vi "WPI_CameraSend Images To PC LoopCustom2.vi"(8 "error in (no error)":errorcluster, 11 "CameraDevRef":T1) -> ()   [LabVIEW 2015]
doc: "This VI is used to send images to the dashboard using the second enet port on the 8 slot controller. This is provided for compatibility, but is higher overhead than using the Camera MJPG approach.\n\nThis software is licensed. Open the labview\\readme\\WPI Robotics Library Open Source License.txt file for more information."
uses:
  <vilib>/Rock Robotics/WPI/Camera/WPI_CameraDevRef.ctl
  <vilib>/Rock Robotics/SystemInterfaces/NetworkCommunication/NetComm_UsageReport_ResourceType.ctl
  Robot Global Data.vi
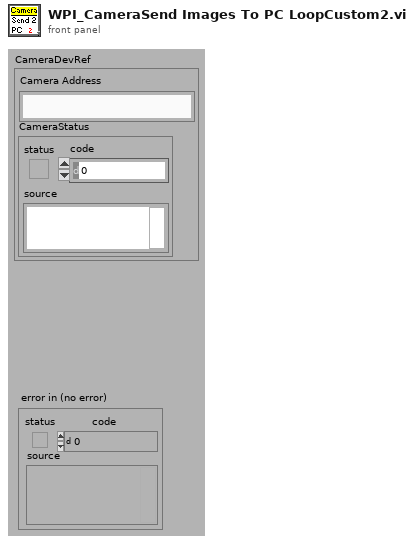
[diagram p1: front panel]
types:
  T1 = typedef "WPI_CameraDevRef.ctl" = cluster{"Camera Address":string, "CameraStatus":errorcluster}
  T2 = cluster{"fps":i32, "compression":i32, "compression 2":i32}
  T3 = typedef "NetComm_UsageReport_ResourceType.ctl" = enum8{"Controller", "Module", "Language", "CANPlugin", "Accelerometer", "ADXL345", "AnalogChannel", "AnalogTrigger", "AnalogTriggerOutput", "CANJaguar", "Compressor", "Counter", "Dashboard", "DigitalInput", "DigitalOutput", "DriverStationCIO", "DriverStationEIO", "DriverStationLCD", "Encoder", "GearTooth", "Gyro", "I2C", "Framework", "Jaguar", "Joystick", "Kinect", "KinectStick", "PIDController", "Preferences", "PWM", "Relay", "RobotDrive", "SerialPort", "Servo", "Solenoid", "SPI", "Task", "Ultrasonic", "Victor", "Button", "Command", "AxisCamera", "PCVideoServer", "SmartDashboard", "Talon", "HiTechnicColorSensor", "HiTechnicAccel", "HiTechnicCompass", "SRF08", "AnalogOutput", "Victor SP", "Talon SRX", "CAN Talon SRX", "ADXL362 Accel", "ADXRS450 Gyro", "Rev SPARK", "Mindsensors SD540", "Digital Filter"}
  T4 = enum16{"Update Mode", "Get Image", "Get Image Data"}
  T5 = typedef "Image Type" = u32
  T6 = typedef "IMAQ Image.ctl" = refnum<image>
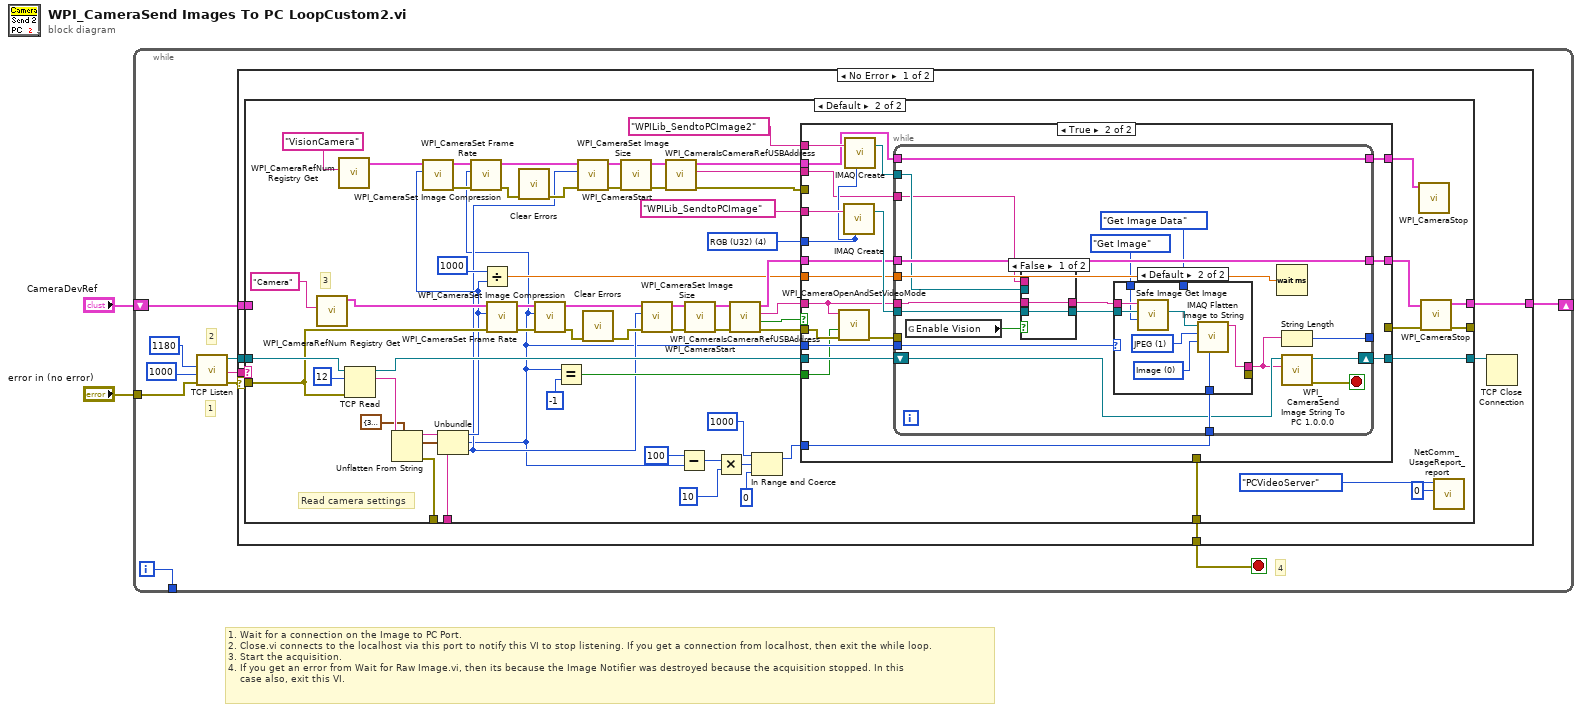
[diagram p0: block diagram]
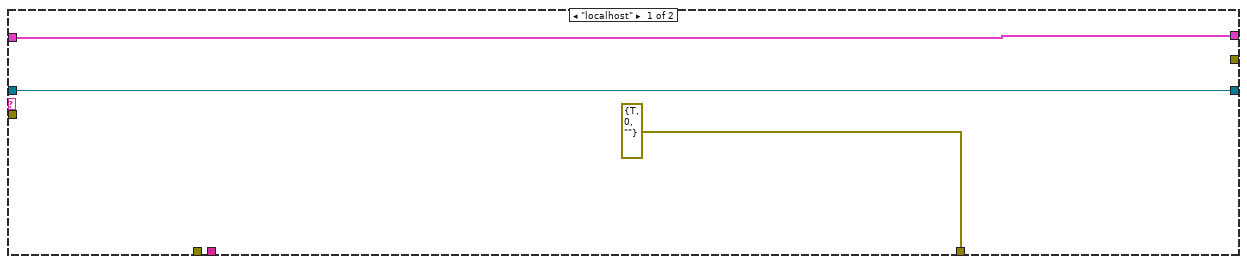
[diagram p2: hidden frame]
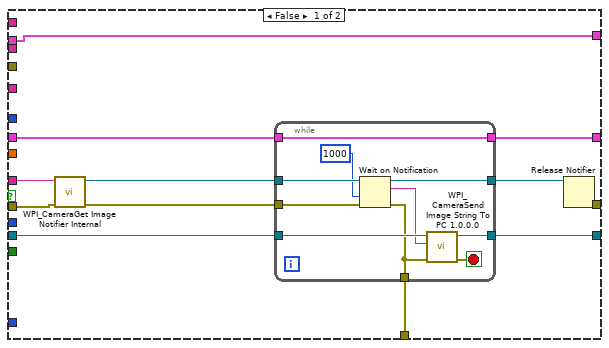
[diagram p3: hidden frame]
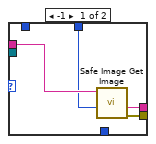
[diagram p5: hidden frame]
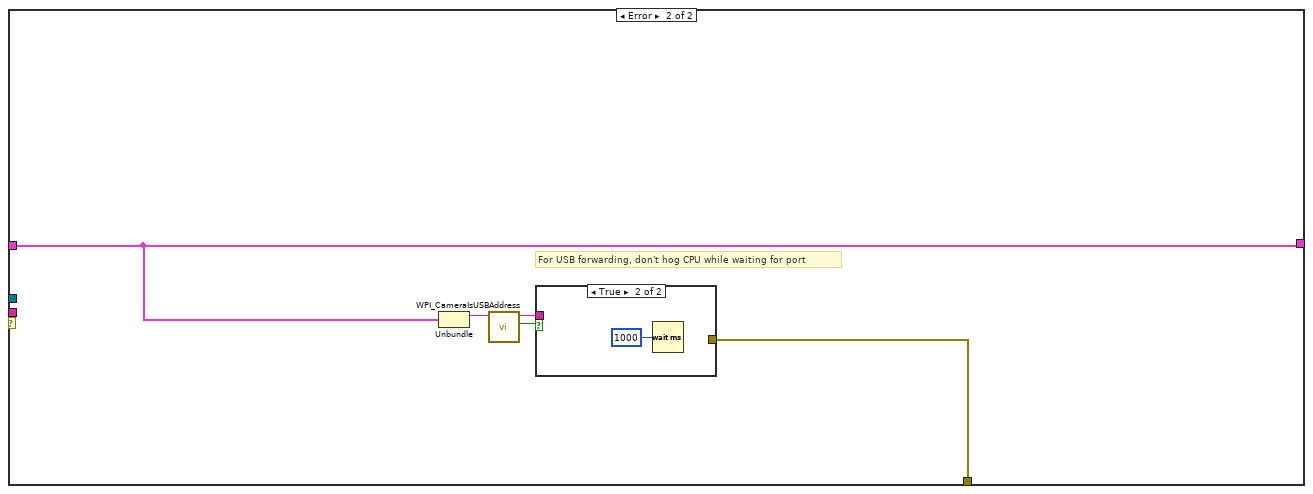
[diagram p6: hidden frame]
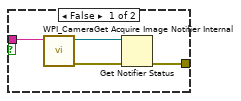
[diagram p7: hidden frame]
diagram:
  # "1. Wait for a connection on the Image to PC Port.\n2. Close.vi connects to the localhost via this port to notify this VI to stop listening. If you get a connection from localhost, then exit the while loop.\n3. Start the acquisition.\n4. If you get an error from Wait for Raw Image.vi, then its because the Image Notifier was destroyed because the acquisition stopped. In this\n    case also, exit this VI."
  n1 = while {
    tunnel: "error in (no error)" -> [w9]
    shift-right: [w12] -> _
    shift-left: "CameraDevRef" -> [w10]
    tunnel: [w3] -> _
    i -> [w3]
    stop <- w7 stop-if-true
    # "4"
    # "1"
    # "2"
    n2 = call <vilib>:"TCP Listen.vi"("error in (no error)"=w9, "timeout ms (wait forever: -1)"=u16 1000 ("port"), "port"=u16 1180) -> ("error out"=w5:errorcluster, "remote address"=w11:string, "connection ID"=w8:refnum<k5>)  [unwired: 1 in, 5 out]
    n3 = case shown="No Error" w5 {
      selector: w5 -> [w13 _]
      tunnel: [w19 w166] -> w12
      tunnel: w11 -> [w18 _]
      tunnel: w10 -> [w17 w166]
      tunnel: w8 -> [w16 _]
      tunnel: [w15 w167] -> w7
      frame No Error {
        n4 = case shown="Default" w18 {
          tunnel: [w22 w84] -> w19
          tunnel: w17 -> [w22 _]
          tunnel: w13 -> [_ w63]
          tunnel: w16 -> [w20 w70]
          tunnel: [errorcluster {"status"=TRUE, "code"=0, "source"=""} ("error out 2") w86] -> w15
          tunnel: [w20 w85] -> w14
          tunnel: [_ w83] -> _
          tunnel: [_ w45] -> _
          tunnel: [_ w44] -> _
          frame "localhost" {
          }
          frame Default {
            w77 = T5 4 items=["Grayscale (U8)", "Grayscale (I16)", "Grayscale (SGL)", "Complex (CSG)", "RGB (U32)", "HSL (U32)", "RGB (U64)", "Grayscale (U16)"] ("Image Type")
            # "Read camera settings"
            # "3"
            n5 = call <vilib>:"WPI_CameraRefNum Registry Get.vi"("refnum name"="Camera") -> ("CameraDevRef"=w41:T1)  [unwired: 9 in, 1 out]
            n6 = call <vilib>:"WPI_CameraRefNum Registry Get.vi"("refnum name"="VisionCamera") -> ("CameraDevRef"=w31:T1)  [unwired: 9 in, 1 out]
            n7 = TCP Read(connection ID=w70, bytes to read=12, error in (no error)=w63) -> (connection ID out=w69:refnum<k5>, data out=w67:string)  [unwired: 2 in, 1 out]
            n8 = Unflatten From String(type=T2 {"fps"=30, "compression"=32, "compression 2"=32} ("Camera Settings"), binary string=w67) -> (rest of the binary string=w44:string, value=w60:T2, error out=w45:errorcluster)  [unwired: 3 in]
            n9 = Unbundle(w60) -> ("fps"=w30:i32, "compression"=w23:i32, "compression 2"=w24:i32)
            n10 = call <vilib>:"WPI_CameraSet Frame Rate.vi"("Frame Rate (fps)"=w30, "CameraDevRef"=w31) -> ("error out"=w37:errorcluster, "CameraDevRef Out"=w34:T1)  [unwired: 8 in]
            n11 = call <vilib>:"WPI_CameraSet Image Compression.vi"("error in (no error)"=w37, "Compression"=w23, "CameraDevRef"=w34) -> ("error out"=w39:errorcluster, "CameraDevRef Out"=w35:T1)  [unwired: 7 in]
            n12 = Divide(x=u16 1000 ("port"), y=w30) -> (x/y=w58:dbl)
            n13 = call <vilib>:"WPI_CameraSet Frame Rate.vi"("error in (no error)"=w63, "Frame Rate (fps)"=w30, "CameraDevRef"=w41) -> ("error out"=w62:errorcluster, "CameraDevRef Out"=w66:T1)  [unwired: 7 in]
            n14 = call <vilib>:"Clear Errors.vi"("error in (no error)"=w39) -> ("error out"=w40:errorcluster)  [unwired: 5 in, 1 out]
            n15 = call <vilib>:"WPI_CameraSet Image Compression.vi"("error in (no error)"=w62, "Compression"=w23, "CameraDevRef"=w66) -> ("error out"=w47:errorcluster, "CameraDevRef Out"=w65:T1)  [unwired: 7 in]
            n16 = Equal?(x=w23, y=-1) -> (x = y?=w48:bool)
            n17 = call <vilib>:"WPI_CameraSet Image Size.vi"("error in (no error)"=w40, "Image Size"=w24, "CameraDevRef"=w35) -> ("error out"=w38:errorcluster, "CameraDevRef Out"=w36:T1)  [unwired: 7 in]
            n18 = call <vilib>:"Clear Errors.vi"("error in (no error)"=w47) -> ("error out"=w46:errorcluster)  [unwired: 5 in, 1 out]
            n19 = call <vilib>:"WPI_CameraStart.vi"("error in (no error)"=w38, "CameraDevRef"=w36) -> ("error out"=w32:errorcluster, "CameraDevRef"=w33:T1)  [unwired: 8 out]
            n20 = call <vilib>:"WPI_CameraSet Image Size.vi"("error in (no error)"=w46, "Image Size"=w24, "CameraDevRef"=w65) -> ("error out"=w61:errorcluster, "CameraDevRef Out"=w64:T1)  [unwired: 7 in]
            n21 = call <vilib>:"WPI_CameraIsCameraRefUSBAddress.vi"("error in (no error)"=w32, "CameraDevRef"=w33) -> ("error out"=w29:errorcluster, "Camera Address Out"=w27:string, "CameraDevRef out"=w26:T1)  [unwired: 6 in, 1 out]
            n22 = Subtract(x=100, y=w23) -> (x-y=w53:i32)
            n23 = call <vilib>:"WPI_CameraStart.vi"("error in (no error)"=w61, "CameraDevRef"=w64) -> ("error out"=w74:errorcluster, "CameraDevRef"=w72:T1)  [unwired: 8 out]
            n24 = Multiply(x=w53, y=10) -> (x*y=w55:i32)
            n25 = call <vilib>:"WPI_CameraIsCameraRefUSBAddress.vi"("error in (no error)"=w74, "CameraDevRef"=w72) -> ("error out"=w73:errorcluster, "USB?"=w75:bool, "Camera Address Out"=w76:string, "CameraDevRef out"=w71:T1)  [unwired: 6 in]
            n26 = In Range and Coerce(upper limit=1000, x=w55, lower limit=0) -> (coerced(x)=w51:i32)  [unwired: 1 out]
            n27 = case shown="True" w75 {
              tunnel: w69 -> [w98 w127]
              tunnel: [w97 _] -> w86
              tunnel: [w96 w126] -> w85
              tunnel: w73 -> [w95 w118]
              tunnel: w76 -> [w93 w117]
              tunnel: [w92 w122] -> w82
              tunnel: w71 -> [w91 w123]
              tunnel: [w89 _] -> w81
              tunnel: "WPILib_SendtoPCImage" -> [_ w124]
              tunnel: w77 -> [_ w113]
              tunnel: w51 -> [_ w121]
              tunnel: w58 -> [_ w120]
              tunnel: w23 -> [_ w119]
              tunnel: w48 -> [_ w115]
              tunnel: w29 -> [_ _]
              tunnel: "WPILib_SendtoPCImage2" -> [_ w114]
              tunnel: w27 -> [_ w111]
              tunnel: w26 -> [w87 w110]
              tunnel: [w87 w109] -> w25
              frame False {
                n28 = call <vilib>:"WPI_CameraGet Image Notifier Internal.vi"("error in (no error)"=w95, "Camera Address"=w93) -> ("error out"=w94:errorcluster, "Image Notifier"=w90:refnum<notifier>)  [unwired: 8 out]
                n29 = while {
                  tunnel: w94 -> [w104]
                  tunnel: w98 -> [w108]
                  tunnel: [w101] -> w97
                  tunnel: [w106] -> w96
                  tunnel: [w105] -> w92
                  tunnel: w91 -> [w105]
                  tunnel: w90 -> [w103]
                  tunnel: [w99] -> w88
                  stop <- w107 stop-if-true
                  n30 = Wait on Notification(notifier=w103, timeout in ms (-1)=1000 ("Timeout in ms (-1)"), error in (no error)=w104) -> (notifier out=w99:refnum<notifier>, notification=w102:string, error out=w101:errorcluster)  [unwired: 2 out]
                  n31 = call <vilib>:"WPI_CameraSend Image String To PC 1.0.0.0.vi"("error in (no error)"=w101, "String"=w102, "TCP Connection ID"=w108) -> ("error out"=w107:errorcluster, "TCP Connection ID out"=w106:refnum<k5>)  [unwired: 7 out]
                }
                n32 = Release Notifier(notifier=w88) -> (error out=w89:errorcluster)  [unwired: 1 in, 3 out]
              }
              frame True {
                n33 = call <vilib>:"WPI_CameraOpenAndSetVideoMode.vi"("error in (no error)"=w118, "USB JPEG"=w115, "Camera Address Out"=w117) -> ("error out"=w116:errorcluster)  [unwired: 8 in]
                n34 = call "IMAQ Create"("Image Name"=w124, "Image Type"=w113) -> ("New Image"=w125:T6)  [unwired: 3 in, 1 out]
                n35 = call "IMAQ Create"("Image Name"=w114, "Image Type"=w113) -> ("New Image"=w112:T6)  [unwired: 3 in, 1 out]
                n36 = while {
                  tunnel: w117 -> [w132]
                  shift-right: [w146] -> w126
                  shift-left: w127 -> [w142]
                  tunnel: w125 -> [w134]
                  tunnel: [w145] -> w122
                  tunnel: w123 -> [w145]
                  tunnel: w121 -> [w144]
                  tunnel: w120 -> [w143]
                  tunnel: [w140] -> _
                  tunnel: w119 -> [w139]
                  tunnel: w116 -> [_]
                  tunnel: w112 -> [w130]
                  tunnel: w111 -> [w129]
                  tunnel: w110 -> [w128]
                  tunnel: [w128] -> w109
                  stop <- w136 stop-if-true
                  n37 = global read "Robot Global Data.vi" "Enable Vision"() -> (w135:bool)
                  n38 = case shown="False" w135 {
                    tunnel: w134 -> [w148 _]
                    tunnel: [w148 w150] -> w133
                    tunnel: w132 -> [w147 _]
                    tunnel: [w147 w149] -> w131
                    tunnel: w130 -> [_ w150]
                    tunnel: w129 -> [_ w149]
                    frame False {
                    }
                    frame True {
                    }
                  }
                  n39 = case shown="Default" w139 {
                    tunnel: [w153 w162] -> w141
                    tunnel: w131 -> [w154 w158]
                    tunnel: w133 -> [_ w157]
                    tunnel: w144 -> [_ w159]
                    tunnel: [w152 _] -> _
                    tunnel: T4."Get Image Data" ("Operation") -> [w151 _]
                    tunnel: T4."Get Image" ("Operation") -> [_ w155]
                    frame -1 {
                      n40 = call <vilib>:"Safe Image Get Image.vi"("Operation"=w151, "Session In"=w154) -> ("error out"=w152:errorcluster, "Image Data String"=w153:string)  [unwired: 6 in, 2 out]
                    }
                    frame Default {
                      w160 = 0 items=["Image", "Image and Vision Info", "Reference to Image"] ("Type of Flatten (Image and Vision Info)")
                      w161 = 1 items=["None", "JPEG", "PACKED BINARY"] ("Compression (None)")
                      n41 = call <vilib>:"Safe Image Get Image.vi"("Operation"=w155, "Image In"=w157, "Session In"=w158) -> ("Image Out"=w156:T6)  [unwired: 5 in, 3 out]
                      n42 = call "IMAQ Flatten Image to String"("Quality (750)"=w159, "Type of Flatten (Image and Vision Info)"=w160, "Compression (None)"=w161, "Image"=w156) -> ("Data String"=w162:string)  [unwired: 6 in, 1 out]
                    }
                  }
                  n43 = Wait (ms)(milliseconds to wait=w143) -> ()  [unwired: 1 out]
                  n44 = String Length(string=w141) -> (length=w140:i32)
                  n45 = call <vilib>:"WPI_CameraSend Image String To PC 1.0.0.0.vi"("String"=w141, "TCP Connection ID"=w142) -> ("error out"=w136:errorcluster, "TCP Connection ID out"=w146:refnum<k5>)  [unwired: 1 in, 7 out]
                }
              }
            }
            n46 = call <vilib>:"WPI_CameraStop.vi"("CameraDevRef"=w25) -> ()  [unwired: 1 in, 10 out]
            n47 = call <vilib>:"WPI_CameraStop.vi"("error in (no error)"=w81, "CameraDevRef"=w82) -> ("error out"=w83:errorcluster, "CameraDevRef"=w84:T1)  [unwired: 8 out]
            n48 = call <vilib>:"NetComm_UsageReport_report.vi"("Instance Number"=u8 0, "Resource Type"=NetComm_UsageReport_ResourceType."PCVideoServer") -> ()  [unwired: 10 in]
          }
        }
        n49 = TCP Close Connection(connection ID=w14) -> ()  [unwired: 1 in, 3 out]
      }
      frame Error {
        # "For USB forwarding, don't hog CPU while waiting for port"
        n50 = Unbundle(w166) -> ("Camera Address"=w165:string)  [unwired: 1 out]
        n51 = call <vilib>:"WPI_CameraIsUSBAddress.vi"("Camera Address In"=w165) -> ("USB?"=w163:bool, "Camera Address Out"=w164:string)  [unwired: 8 in, 1 out]
        n52 = case shown="True" w163 {
          tunnel: [w171 _] -> w167
          tunnel: w164 -> [w168 _]
          frame False {
            n53 = call <vilib>:"WPI_CameraGet Acquire Image Notifier Internal.vi"("Camera Address"=w168) -> ("error out"=w169:errorcluster, "Acquire Image Notifier"=w170:refnum<notifier>)  [unwired: 1 in, 8 out]
            n54 = Get Notifier Status(notifier=w170, error in (no error)=w169) -> (error out=w171:errorcluster)  [unwired: 4 out]
          }
          frame True {
            n55 = Wait (ms)(milliseconds to wait=u32 1000) -> ()  [unwired: 1 out]
          }
        }
      }
    }
  }
